vi "Dev_code.vi"() -> ()   [LabVIEW 2021]
panel:
  out "Logic Sequence":string
  out "Configuration":string
  in  "Filtered Config Entries":string="1737340154015584000\ttest\tCreate\tTemplatePlugin.0.2.3.lvlibp:TemplatePlugin.lvclass\t<version> 0.2.3.0\t\n1737340198541890000\ttest\tConfigure\t{\"Common\":{\"Period (s)\":0.001,\"Offset (us)\":0,\"ClockID\":0,\"Priority\":101,\"Processor\":-2},\"Step\":100}\n1737340326509796000\tlovingit6\tCreate\tCIFCorePlugin.0.1.2.lvlibp:CIFCorePlugin.lvclass\t<version> 0.1.2.0\t\n1737340326559504000\tchannelme\tCreate\tTemplatePlugin.0.2.3.lvlibp:TemplatePlugin.lvclass\t<version> 0.2.3.0\t\n1737340326827852000\tchannelme\tConnect\t<publisher> channelme/doubleout <subscriber> channelme/doublein1 <data> \n1737340326835711000\tchannelme\tConfigure\t{\"Common\":{\"Period (s)\":0.001,\"Offset (us)\":0,\"ClockID\":0,\"Priority\":101,\"Processor\":-2},\"Step\":100}\n1737340327017380000\tlovingit6\tRun\n"
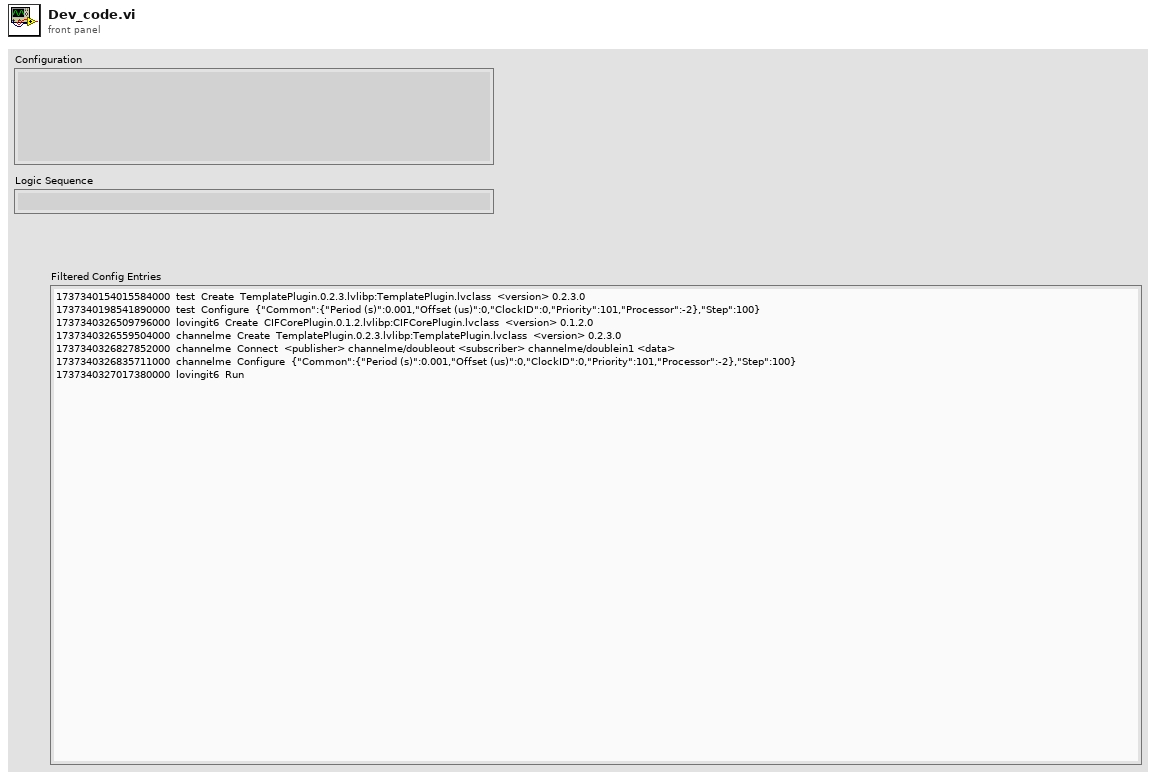
[diagram p1: front panel]
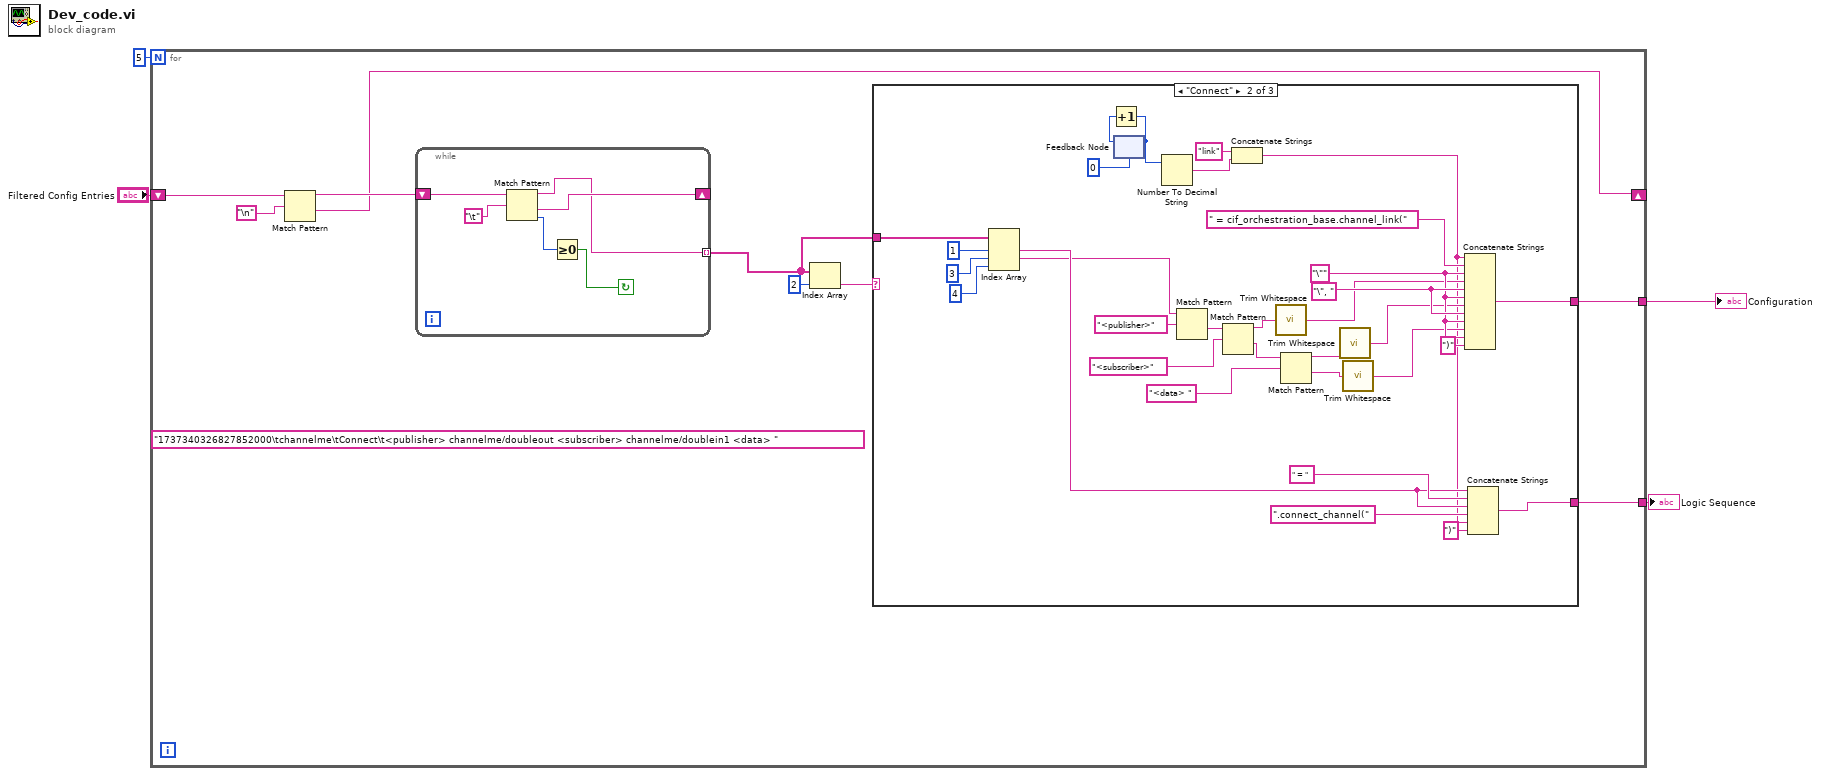
[diagram p0: block diagram]
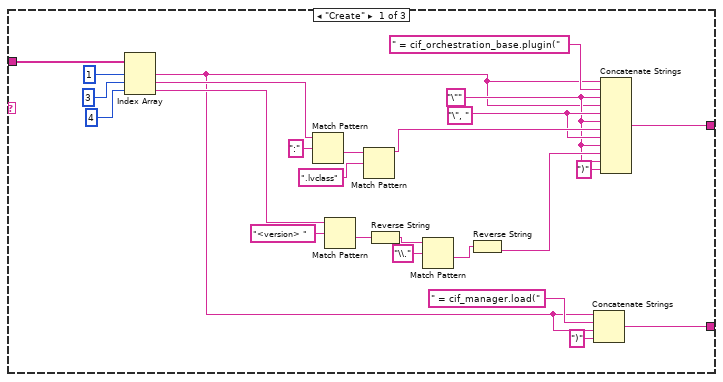
[diagram p2: hidden frame]
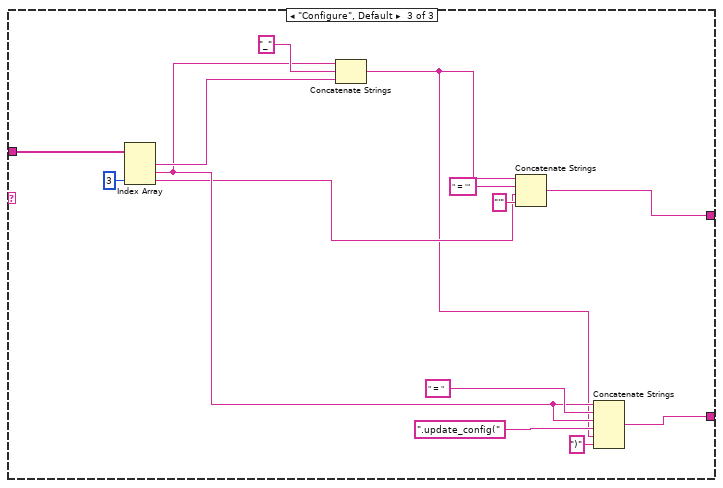
[diagram p3: hidden frame]
diagram:
  n1 = for {
    N: 5 -> [_]
    tunnel: [w7] -> w3
    tunnel: [w6] -> w2
    shift-right: [w5] -> _
    shift-left: "Filtered Config Entries" -> [w13]
    (unwired) "1737340326827852000\tchannelme\tConnect\t<publisher> channelme/doubleout <subscriber> channelme/doublein1 <data> "
    n2 = Match Pattern(string=w13, regular expression="\n") -> (before substring=w11:string, after substring=w5:string)  [unwired: 1 in, 2 out]
    n3 = while {
      shift-right: [w88] -> _
      shift-left: w11 -> [w90]
      tunnel: [w87] -> w10 mode=indexing
      stop <- w85 continue-if-true
      n4 = Match Pattern(string=w90, regular expression="\t") -> (before substring=w87:string, after substring=w88:string, offset past match=w86:i32)  [unwired: 1 in, 1 out]
      n5 = Greater Or Equal To 0?(x=w86) -> (x >= 0?=w85:bool)
    }
    n6 = Index Array(array=w10, index=2) -> (element=w9:string)
    n7 = case shown="\"Connect\"" w9 {
      tunnel: w10 -> [w38 w70 w84]
      tunnel: [w18 w60 w72] -> w7
      tunnel: [w14 w56 w81] -> w6
      frame "Create" {
        w29 = "\", "
        w20 = "\""
        n8 = Index Array(array=w38, index #1=1 ("index"), index #2=3 ("index"), index #3=4 ("index")) -> (element #1=w16:string, element #2=w34:string, element #3=w27:string)
        n9 = Match Pattern(string=w34, regular expression=":") -> (after substring=w32:string)  [unwired: 1 in, 3 out]
        n10 = Match Pattern(string=w27, regular expression="<version> ") -> (after substring=w25:string)  [unwired: 1 in, 3 out]
        n11 = Match Pattern(string=w32, regular expression=".lvclass") -> (before substring=w30:string)  [unwired: 1 in, 3 out]
        n12 = Reverse String(1:w25) -> (0:w24:string)
        n13 = Match Pattern(string=w24, regular expression="\\.") -> (after substring=w22:string)  [unwired: 1 in, 3 out]
        n14 = Reverse String(1:w22) -> (0:w21:string)
        n15 = Concatenate Strings(w16, " = cif_manager.load(", w16, ")" ("string")) -> (w14:string)
        n16 = Concatenate Strings(w16, " = cif_orchestration_base.plugin(", w20, w16, w29, w20, w30, w29, w20, w21, w20, ")" ("string")) -> (w18:string)
      }
      frame "Connect" {
        w64 = "\", "
        w62 = "\""
        n17 = Index Array(array=w70, index #1=1 ("index"), index #2=3 ("index"), index #3=4 ("index")) -> (element #1=w58:string, element #2=w50:string)  [unwired: 1 out]
        n18 = feedback #1(u16 0) -> (w54:u16)
        n19 = Increment(x=w54) -> (x+1=w53:u16)
        n20 = feedback-in #1(w53) -> ()
        n21 = Number To Decimal String(number=w53) -> (decimal integer string=w51:string)  [unwired: 1 in]
        n22 = Match Pattern(string=w50, regular expression="<publisher>") -> (after substring=w65:string)  [unwired: 1 in, 3 out]
        n23 = Match Pattern(string=w65, regular expression="<subscriber>") -> (before substring=w48:string, after substring=w46:string)  [unwired: 1 in, 2 out]
        n24 = Concatenate Strings("link" ("string"), w51) -> (w40:string)
        n25 = call <vilib>:"Trim Whitespace.vi"("string"=w48) -> ("trimmed string"=w47:string)  [unwired: 1 in]
        n26 = Match Pattern(string=w46, regular expression="<data> ") -> (before substring=w44:string, after substring=w42:string)  [unwired: 1 in, 2 out]
        n27 = call <vilib>:"Trim Whitespace.vi"("string"=w44) -> ("trimmed string"=w43:string)  [unwired: 1 in]
        n28 = call <vilib>:"Trim Whitespace.vi"("string"=w42) -> ("trimmed string"=w41:string)  [unwired: 1 in]
        n29 = Concatenate Strings(w40, " = cif_orchestration_base.channel_link(", w62, w47, w64, w62, w43, w64, w62, w41, w62, ")" ("string")) -> (w60:string)
        n30 = Concatenate Strings(w58, " = ", w58, ".connect_channel(" ("string"), w40, ")" ("string")) -> (w56:string)
      }
      frame "Configure", Default {
        n31 = Index Array(array=w84, index #3=3 ("index")) -> (element #1=w79:string, element #2=w77:string, element #3=w73:string)  [unwired: 2 in]
        n32 = Concatenate Strings(w77, "_" ("string"), w79) -> (w71:string)
        n33 = Concatenate Strings(w71, " = '" ("string"), w73, "'" ("string")) -> (w72:string)
        n34 = Concatenate Strings(w77, " = ", w77, ".update_config(" ("string"), w71, ")" ("string")) -> (w81:string)
      }
    }
  }
  "Configuration" <- w3
  "Logic Sequence" <- w2
